vi "Scripting_FollowWireUpStream.vi"(0 "Scripting in":refnum<class "Scripting.lvclass">, 1 "StartTerminalRef":refnum<vi>, 5 "error in (no error)":errorcluster) -> (15 "FoundItems":T1[](array[typedef]), 19 "error out":errorcluster)   [LabVIEW 2016, in "Scripting.lvclass"]
uses:
  <resource>/Framework/Providers/Open_GDS/ClassProviders/Common/ScriptingFunctions/Scripting.lvclass
  <resource>/Framework/Providers/Open_GDS/ClassProviders/Common/ScriptingFunctions/Scripting_PastThroughObjectType.ctl
  <resource>/Framework/Providers/Open_GDS/ClassProviders/Common/ScriptingFunctions/Scripting_ObjectType.ctl
  <resource>/Framework/Providers/Open_GDS/ClassProviders/Common/ScriptingFunctions/Scripting.lvclass/Scripting.ctl
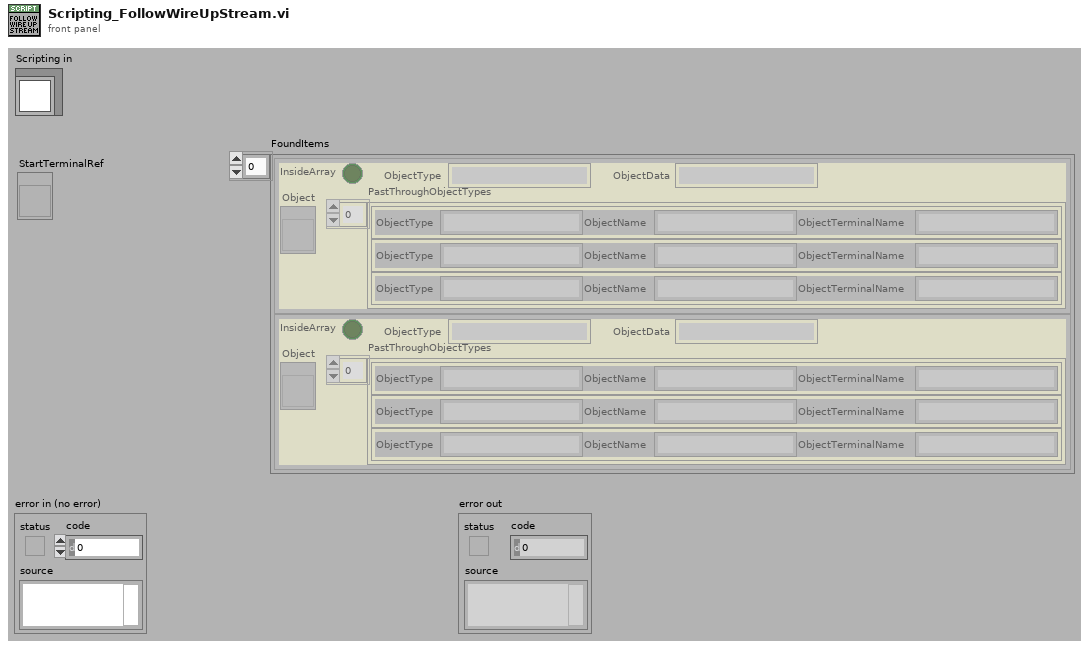
[diagram p1: front panel]
types:
  T1 = typedef "Scripting.lvclass/Scripting_PastThroughObjectType.ctl" = cluster{"Object":refnum<vi>, "InsideArray":bool, "PastThroughObjectTypes":T2[], "ObjectType":string, "ObjectData":string}
  T2 = typedef "Scripting_ObjectType.ctl" = cluster{"ObjectType":string, "ObjectName":string, "ObjectTerminalName":string}
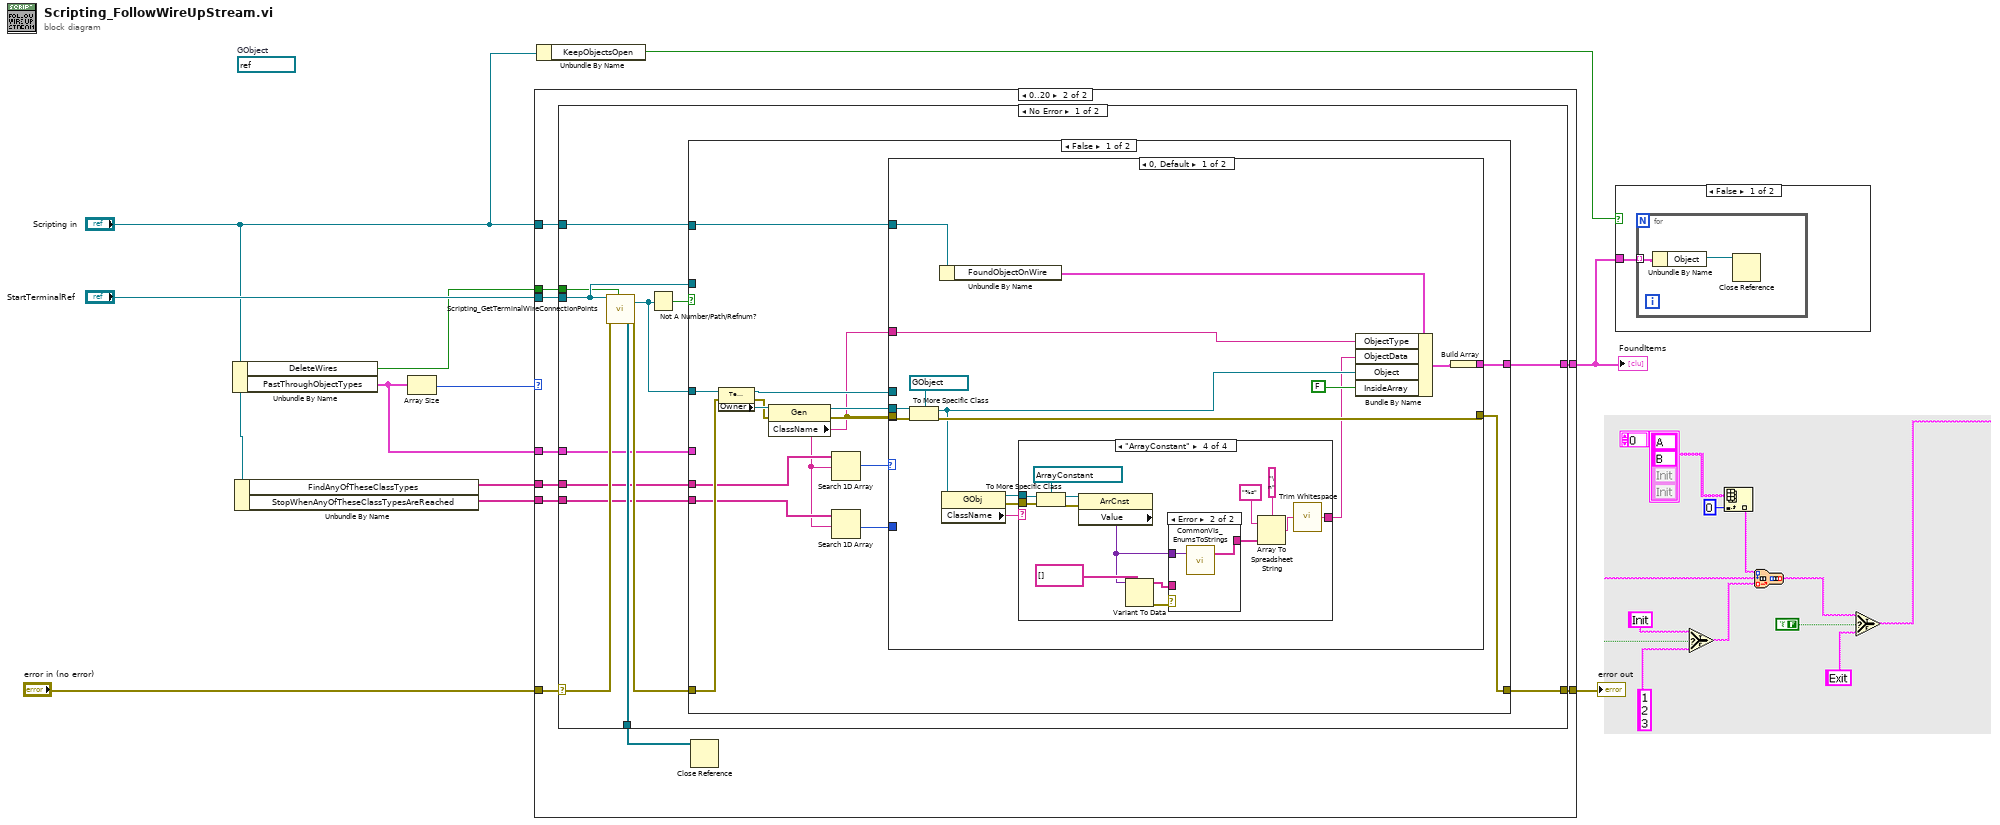
[diagram p0: block diagram]
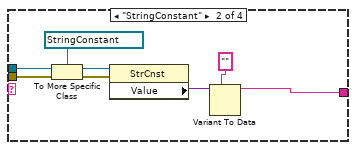
[diagram p5: hidden frame]
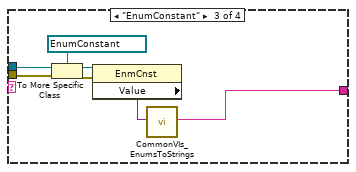
[diagram p6: hidden frame]
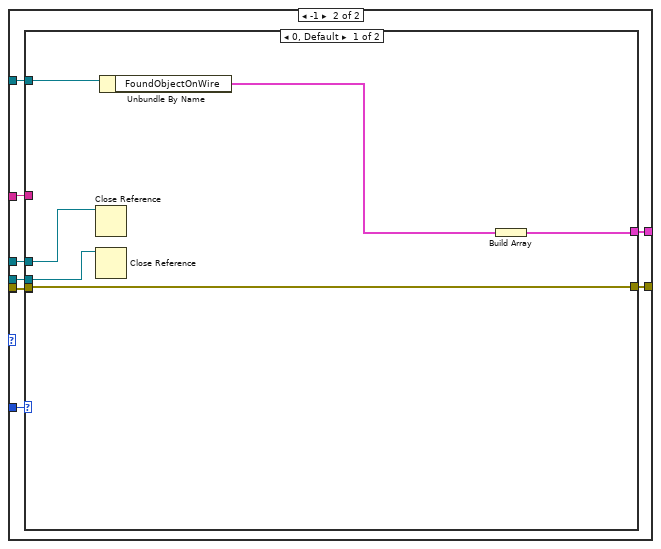
[diagram p8: hidden frame]
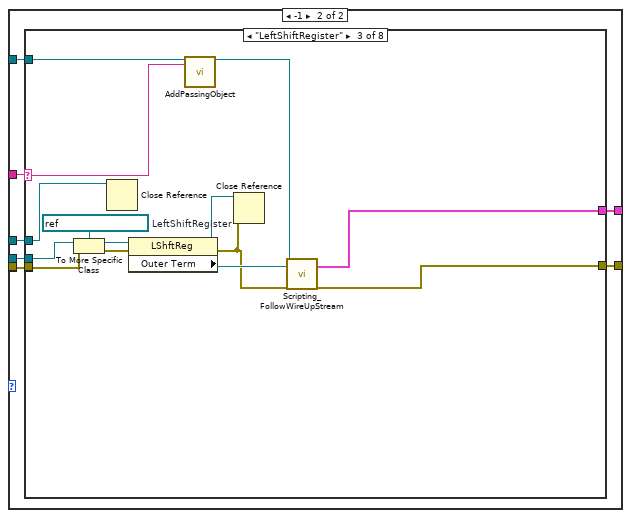
[diagram p9: hidden frame]
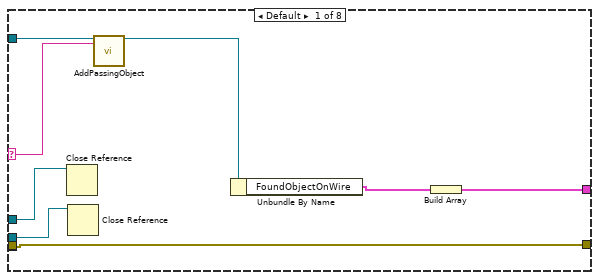
[diagram p10: hidden frame]
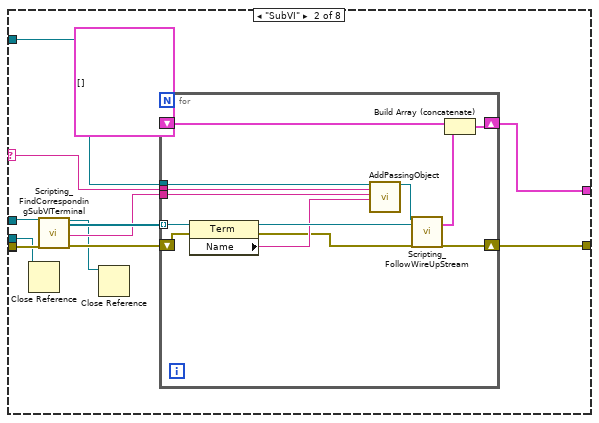
[diagram p11: hidden frame]
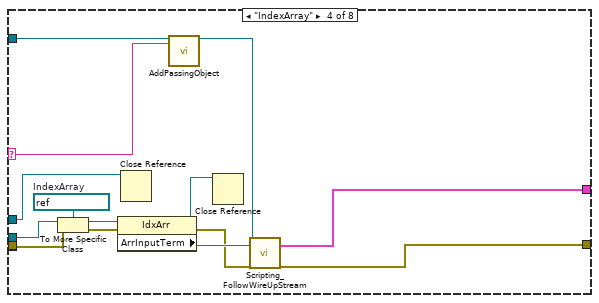
[diagram p12: hidden frame]
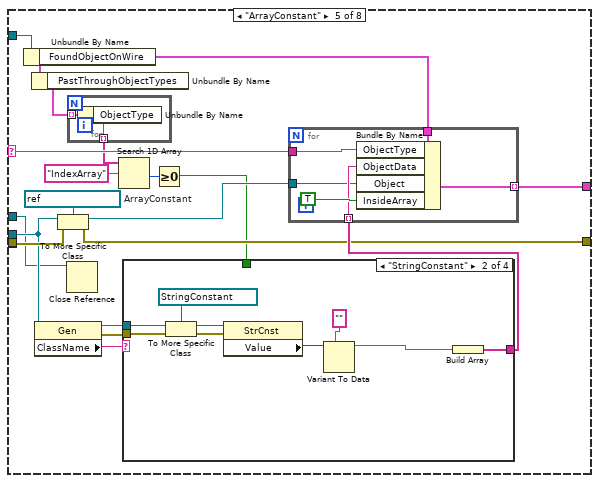
[diagram p13: hidden frame]
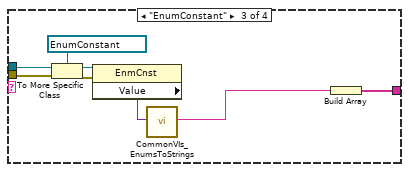
[diagram p15: hidden frame]
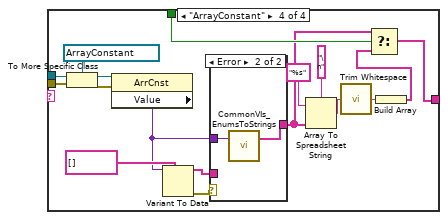
[diagram p16: hidden frame]
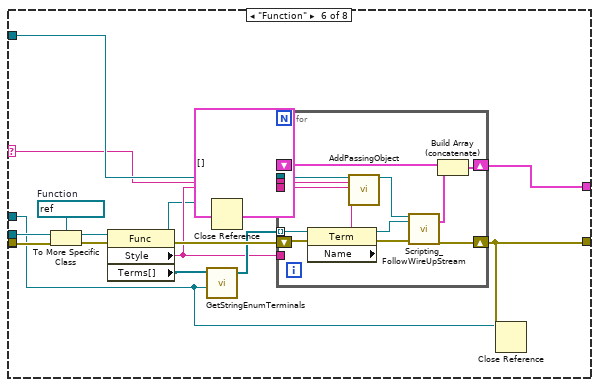
[diagram p18: hidden frame]
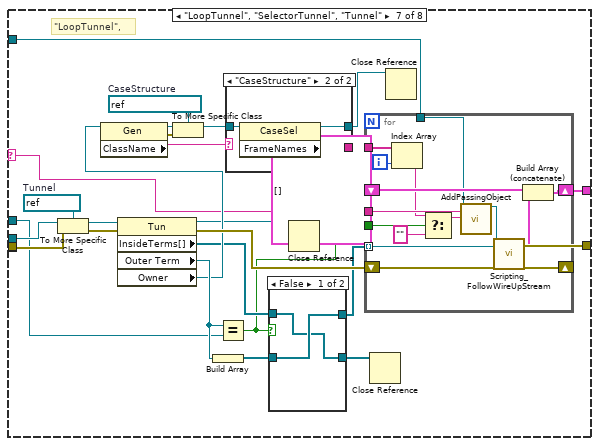
[diagram p19: hidden frame]
diagram:
  (unwired) refnum<vi> refnum  # GObject
  n1 = Unbundle By Name("Scripting in") -> ("DeleteWires"=w1:bool, "PastThroughObjectTypes"=w5:T2[])
  n2 = Unbundle By Name("Scripting in") -> ("FindAnyOfTheseClassTypes"=w8:string[], "StopWhenAnyOfTheseClassTypesAreReached"=w7:string[])
  n3 = Array Size(array=w5) -> (size(s)=w6:i32)
  n4 = case shown="0..20" w6 {
    tunnel: [w12 w22] -> w11
    tunnel: "error in (no error)" -> [w12 w21]
    tunnel: "StartTerminalRef" -> [_ w20]
    tunnel: w8 -> [_ w18]
    tunnel: w7 -> [_ w17]
    tunnel: [_ w16] -> w4
    tunnel: "Scripting in" -> [_ w15]
    tunnel: w5 -> [_ w14]
    tunnel: w1 -> [_ w13]
    frame Default {
    }
    frame 0..20 {
      n5 = case shown="No Error" w21 {
        selector: w21 -> [w31 w369]
        tunnel: [w33 w369] -> w22
        tunnel: w15 -> [w29 _]
        tunnel: w20 -> [w25 _]
        tunnel: [w35 _] -> w19
        tunnel: w18 -> [w28 _]
        tunnel: w17 -> [w27 _]
        tunnel: [w26 _] -> w16
        tunnel: w14 -> [w24 _]
        tunnel: w13 -> [w23 _]
        frame No Error {
          n6 = call <resource>:"Scripting_GetTerminalWireConnectionPoints.vi"("Term Refnum In"=w25, "error in"=w31, "RemoveWire(False)"=w23) -> ("AllWireTerminals"=w35:refnum<vi>[], "WireTermSource"=w32:refnum<vi>, "error out"=w30:errorcluster)  [unwired: 8 in, 6 out]
          n7 = Not A Number/Path/Refnum?(number/path/refnum=w32) -> (NaN/Path/Refnum?=w34:bool)
          n8 = case shown="False" w34 {
            tunnel: w30 -> [w49 w360]
            tunnel: [w47 w360] -> w33
            tunnel: w32 -> [w50 _]
            tunnel: w29 -> [w48 w355]
            tunnel: w28 -> [w46 _]
            tunnel: w27 -> [w45 _]
            tunnel: [w37 w352] -> w26
            tunnel: w25 -> [_ w354]
            tunnel: w24 -> [_ w359]
            frame False {
              n9 = property class="Term"(reference=w50, error in=w49) -> (reference out=w38:refnum<vi>, error out=w41:errorcluster, "Owner"=w42:refnum<vi>)
              n10 = property class="Gen"(reference=w42, error in=w41) -> (reference out=w39:refnum<vi>, error out=w40:errorcluster, "ClassName"=w36:string)
              n11 = Search 1D Array(1D array=w46, element=w36) -> (index of element=w44:i32)  [unwired: 1 in]
              n12 = Search 1D Array(1D array=w45, element=w36) -> (index of element=w43:i32)  [unwired: 1 in]
              n13 = case shown="0, Default" w44 {
                tunnel: w48 -> [w61 w106]
                tunnel: [w62 w105] -> w47
                tunnel: w36 -> [w56 w104]
                tunnel: w43 -> [_ w103]
                tunnel: w40 -> [w65 w102]
                tunnel: w40 -> [_ w101]
                tunnel: w39 -> [w64 w99]
                tunnel: w38 -> [_ w100]
                tunnel: [w57 w98] -> w37
                frame 0, Default {
                  n14 = To More Specific Class(target class=refnum<vi> refnum ("Object"), reference=w64, error in=w65) -> (specific class reference=w55:refnum<vi>, error out=w62:errorcluster)
                  n15 = Unbundle By Name(w61) -> ("FoundObjectOnWire"=w60:T1)
                  n16 = property class="GObj"(reference=w55) -> (reference out=w53:refnum<vi>, error out=w52:errorcluster, "ClassName"=w54:string)  [unwired: 1 in]
                  n17 = case shown="\"ArrayConstant\"" w54 {
                    tunnel: w53 -> [_ w72 w76 w87]
                    tunnel: w52 -> [_ w71 w75 w86]
                    tunnel: [_ w66 w74 w81] -> w51
                    frame Default {
                    }
                    frame "StringConstant" {
                      n18 = To More Specific Class(target class=refnum<vi> refnum ("Object"), reference=w72, error in=w71) -> (specific class reference=w70:refnum<vi>, error out=w69:errorcluster)
                      n19 = property class="StrCnst"(reference=w70, error in=w69) -> ("Value"=w68:variant)  [unwired: 2 out]
                      n20 = Variant To Data(type="" ("Class Name"), Variant=w68) -> (data=w66:string)  [unwired: 1 in, 1 out]
                    }
                    frame "EnumConstant" {
                      n21 = To More Specific Class(target class=refnum<vi> refnum ("WhileLoop"), reference=w76, error in=w75) -> (specific class reference=w79:refnum<vi>, error out=w78:errorcluster)
                      n22 = property class="EnmCnst"(reference=w79, error in=w78) -> ("Value"=w77:variant)  [unwired: 2 out]
                      n23 = call <resource>:"CommonVIs_EnumsToStrings.vi"("SingleEnumVariantIn"=w77) -> ("EnumItem"=w74:string)  [unwired: 2 in, 16 out]
                    }
                    frame "ArrayConstant" {
                      n24 = To More Specific Class(target class=refnum<vi> refnum ("WhileLoop"), reference=w87, error in=w86) -> (specific class reference=w93:refnum<vi>, error out=w92:errorcluster)
                      n25 = property class="ArrCnst"(reference=w93, error in=w92) -> ("Value"=w89:variant)  [unwired: 2 out]
                      n26 = Variant To Data(type=string[] [], Variant=w89) -> (data=w88:string[], error out=w90:errorcluster)  [unwired: 1 in]
                      n27 = case shown="Error" w90 {
                        tunnel: w89 -> [_ w97]
                        tunnel: w88 -> [w95 _]
                        tunnel: [w95 w96] -> w85
                        frame No Error {
                        }
                        frame Error {
                          n28 = call <resource>:"CommonVIs_EnumsToStrings.vi"("ArrayEnumVariantIn"=w97) -> ("EnumItems(string)"=w96:string[])  [unwired: 2 in, 16 out]
                        }
                      }
                      n29 = Array To Spreadsheet String(delimiter (Tab)="\n", array=w85, 3:"%s" ("format string")) -> (spreadsheet string=w82:string)
                      n30 = call <vilib>:"Trim Whitespace.vi"("string"=w82) -> ("trimmed string"=w81:string)  [unwired: 1 in]
                    }
                  }
                  n31 = Bundle By Name(cluster=w60, "ObjectType"=w56, "ObjectData"=w51, "Object"=w55, "InsideArray"=FALSE) -> (w58:T1)
                  n32 = Build Array(w58) -> (w57:T1[])
                }
                frame -1 {
                  n33 = case shown="0, Default" w103 {
                    tunnel: w106 -> [w109 w120]
                    tunnel: [w112 w119] -> w105
                    tunnel: w104 -> [_ w118]
                    tunnel: w102 -> [w112 w117]
                    tunnel: w101 -> [_ w116]
                    tunnel: w100 -> [w111 w115]
                    tunnel: w99 -> [w110 w114]
                    tunnel: [w107 w113] -> w98
                    frame 0, Default {
                      n34 = Close Reference(reference=w111) -> ()  [unwired: 1 in, 1 out]
                      n35 = Close Reference(reference=w110) -> ()  [unwired: 1 in, 1 out]
                      n36 = Unbundle By Name(w109) -> ("FoundObjectOnWire"=w108:T1)
                      n37 = Build Array(w108) -> (w107:T1[])
                    }
                    frame -1 {
                      n38 = case shown="\"LeftShiftRegister\"" w118 {
                        selector: w118 -> [w126 w132 w157 w169 w190 w249 w281 w332]
                        tunnel: w120 -> [w127 w133 w159 w171 w192 w250 w282 w333]
                        tunnel: [w128 w140 w162 w174 w188 w246 w296 w338] -> w119
                        tunnel: w117 -> [w128 _ w166 w180 w199 w260 w300 w341]
                        tunnel: w116 -> [_ w137 _ _ _ _ _ _]
                        tunnel: w115 -> [w125 w136 w153 w167 w181 w245 w290 w331]
                        tunnel: w114 -> [w124 w129 w161 w173 w193 w256 w295 w337]
                        tunnel: [w121 w134 w160 w172 w197 w254 w293 w335] -> w113
                        frame Default {
                          n39 = Close Reference(reference=w125) -> ()  [unwired: 1 in, 1 out]
                          n40 = Close Reference(reference=w124) -> ()  [unwired: 1 in, 1 out]
                          n41 = call <resource>:"AddPassingObject.vi"("object in"=w127, "PassingThroughObject"=w126) -> ("object out"=w123:refnum<class "Scripting.lvclass">)  [unwired: 16 in, 1 out]
                          n42 = Unbundle By Name(w123) -> ("FoundObjectOnWire"=w122:T1)
                          n43 = Build Array(w122) -> (w121:T1[])
                        }
                        frame "SubVI" {
                          n44 = Close Reference(reference=w129) -> ()  [unwired: 1 in, 1 out]
                          n45 = call <resource>:"Scripting_FindCorrespondingSubVITerminal.vi"("SubVITerminalIn"=w136, "error in"=w137) -> ("SubVITerminalIn Dub"=w130:refnum<vi>, "SubVITerminalOut"=w138:refnum<vi>[], "VI Name"=w131:string, "error out"=w139:errorcluster)  [unwired: 11 in, 3 out]
                          n46 = Close Reference(reference=w130) -> ()  [unwired: 1 in, 1 out]
                          n47 = for {
                            tunnel: w138 -> [w143] mode=indexing
                            shift-right: [w152] -> w140
                            shift-left: w139 -> [w144]
                            shift-right: [w150] -> w134
                            shift-left: T1[] [] ("FoundItems") -> [w151]
                            tunnel: w133 -> [w148]
                            tunnel: w132 -> [w146]
                            tunnel: w131 -> [w145]
                            n48 = property class="Term"(reference=w143, error in=w144) -> (error out=w141:errorcluster, "Name"=w142:string)  [unwired: 1 out]
                            n49 = call <resource>:"AddPassingObject.vi"("object in"=w148, "PassingThroughObject"=w146, "PassingThroughObjectName"=w145, "TerminalName"=w142) -> ("object out"=w147:refnum<class "Scripting.lvclass">)  [unwired: 14 in, 1 out]
                            n50 = call-dynamic "Scripting_FollowWireUpStream.vi"("Scripting in"=w147, "StartTerminalRef"=w143, "error in (no error)"=w141) -> ("FoundItems"=w149:T1[], "error out"=w152:errorcluster)  [unwired: 15 in]
                            n51 = Build Array (concatenate)(w151, w149) -> (w150:T1[])
                          }
                        }
                        frame "LeftShiftRegister" {
                          w165 = refnum<vi> refnum  # LeftShiftRegister
                          n52 = To More Specific Class(target class=w165, reference=w161, error in=w166) -> (specific class reference=w154:refnum<vi>, error out=w163:errorcluster)
                          n53 = Close Reference(reference=w153) -> ()  [unwired: 1 in, 1 out]
                          n54 = property class="LShftReg"(reference=w154, error in=w163) -> (reference out=w156:refnum<vi>, error out=w155:errorcluster, "Outer Term"=w164:refnum<vi>)
                          n55 = call <resource>:"AddPassingObject.vi"("object in"=w159, "PassingThroughObject"=w157) -> ("object out"=w158:refnum<class "Scripting.lvclass">)  [unwired: 16 in, 1 out]
                          n56 = Close Reference(reference=w156, error in (no error)=w155) -> ()  [unwired: 1 out]
                          n57 = call-dynamic "Scripting_FollowWireUpStream.vi"("Scripting in"=w158, "StartTerminalRef"=w164, "error in (no error)"=w155) -> ("FoundItems"=w160:T1[], "error out"=w162:errorcluster)  [unwired: 15 in]
                        }
                        frame "IndexArray" {
                          w179 = refnum<vi> refnum  # IndexArray
                          n58 = To More Specific Class(target class=w179, reference=w173, error in=w180) -> (specific class reference=w178:refnum<vi>, error out=w176:errorcluster)
                          n59 = property class="IdxArr"(reference=w178, error in=w176) -> (reference out=w168:refnum<vi>, error out=w175:errorcluster, "ArrInputTerm"=w177:refnum<vi>)
                          n60 = Close Reference(reference=w167) -> ()  [unwired: 1 in, 1 out]
                          n61 = call <resource>:"AddPassingObject.vi"("object in"=w171, "PassingThroughObject"=w169) -> ("object out"=w170:refnum<class "Scripting.lvclass">)  [unwired: 16 in, 1 out]
                          n62 = Close Reference(reference=w168) -> ()  [unwired: 1 in, 1 out]
                          n63 = call-dynamic "Scripting_FollowWireUpStream.vi"("Scripting in"=w170, "StartTerminalRef"=w177, "error in (no error)"=w175) -> ("FoundItems"=w172:T1[], "error out"=w174:errorcluster)  [unwired: 15 in]
                        }
                        frame "ArrayConstant" {
                          w198 = refnum<vi> refnum  # ArrayConstant
                          n64 = Unbundle By Name(w192) -> ("FoundObjectOnWire"=w187:T1)
                          n65 = Unbundle By Name(w187) -> ("PastThroughObjectTypes"=w186:T2[])
                          n66 = property class="Gen"(reference=w193) -> (reference out=w195:refnum<vi>, error out=w194:errorcluster, "ClassName"=w196:string)  [unwired: 1 in]
                          n67 = To More Specific Class(target class=w198, reference=w193, error in=w199) -> (specific class reference=w189:refnum<vi>, error out=w188:errorcluster)
                          n68 = Close Reference(reference=w181) -> ()  [unwired: 1 in, 1 out]
                          n69 = for {
                            tunnel: w186 -> [w201] mode=indexing
                            tunnel: [w200] -> w185 mode=indexing
                            n70 = Unbundle By Name(w201) -> ("ObjectType"=w200:string)
                          }
                          n71 = Search 1D Array(1D array=w185, element="IndexArray") -> (index of element=w183:i32)  [unwired: 1 in]
                          n72 = Greater Or Equal To 0?(x=w183) -> (x >= 0?=w182:bool)
                          n73 = case shown="\"StringConstant\"" w196 {
                            tunnel: w195 -> [_ w215 w220 w234]
                            tunnel: w194 -> [_ w214 w219 w233]
                            tunnel: [_ w208 w217 w225] -> w191
                            tunnel: w182 -> [_ _ _ w228]
                            frame Default {
                            }
                            frame "StringConstant" {
                              n74 = To More Specific Class(target class=refnum<vi> refnum ("Object"), reference=w215, error in=w214) -> (specific class reference=w213:refnum<vi>, error out=w212:errorcluster)
                              n75 = property class="StrCnst"(reference=w213, error in=w212) -> ("Value"=w211:variant)  [unwired: 2 out]
                              n76 = Variant To Data(type="" ("Class Name"), Variant=w211) -> (data=w209:string)  [unwired: 1 in, 1 out]
                              n77 = Build Array(w209) -> (w208:string[])
                            }
                            frame "EnumConstant" {
                              n78 = To More Specific Class(target class=refnum<vi> refnum ("WhileLoop"), reference=w220, error in=w219) -> (specific class reference=w223:refnum<vi>, error out=w222:errorcluster)
                              n79 = property class="EnmCnst"(reference=w223, error in=w222) -> ("Value"=w221:variant)  [unwired: 2 out]
                              n80 = call <resource>:"CommonVIs_EnumsToStrings.vi"("SingleEnumVariantIn"=w221) -> ("EnumItem"=w218:string)  [unwired: 2 in, 16 out]
                              n81 = Build Array(w218) -> (w217:string[])
                            }
                            frame "ArrayConstant" {
                              n82 = To More Specific Class(target class=refnum<vi> refnum ("WhileLoop"), reference=w234, error in=w233) -> (specific class reference=w240:refnum<vi>, error out=w239:errorcluster)
                              n83 = property class="ArrCnst"(reference=w240, error in=w239) -> ("Value"=w236:variant)  [unwired: 2 out]
                              n84 = Variant To Data(type=string[] [], Variant=w236) -> (data=w235:string[], error out=w237:errorcluster)  [unwired: 1 in]
                              n85 = case shown="Error" w237 {
                                tunnel: w236 -> [_ w244]
                                tunnel: w235 -> [w242 _]
                                tunnel: [w242 w243] -> w227
                                frame No Error {
                                }
                                frame Error {
                                n86 = call <resource>:"CommonVIs_EnumsToStrings.vi"("ArrayEnumVariantIn"=w244) -> ("EnumItems(string)"=w243:string[])  [unwired: 2 in, 16 out]
                                }
                              }
                              n87 = Array To Spreadsheet String(delimiter (Tab)="\n", array=w227, 3:"%s" ("format string")) -> (spreadsheet string=w230:string)
                              n88 = call <vilib>:"Trim Whitespace.vi"("string"=w230) -> ("trimmed string"=w229:string)  [unwired: 1 in]
                              n89 = Build Array(w229) -> (w226:string[])
                              n90 = Select(t=w227, s=w228, f=w226) -> (s? t:f=w225:string[])
                            }
                          }
                          n91 = for {
                            tunnel: w187 -> [w207]
                            tunnel: [w202] -> w197 mode=indexing
                            tunnel: w191 -> [w205] mode=indexing
                            tunnel: w190 -> [w204]
                            tunnel: w189 -> [w203]
                            n92 = Bundle By Name(cluster=w207, "ObjectType"=w204, "ObjectData"=w205, "Object"=w203, "InsideArray"=TRUE) -> (w202:T1)
                          }
                        }
                        frame "Function" {
                          w259 = refnum<vi> refnum  # Function
                          n93 = To More Specific Class(target class=w259, reference=w256, error in=w260) -> (specific class reference=w258:refnum<vi>, error out=w257:errorcluster)
                          n94 = property class="Func"(reference=w258, error in=w257) -> (reference out=w247:refnum<vi>, error out=w253:errorcluster, "Style"=w248:string, "Terms[]"=w251:refnum<vi>[])
                          n95 = call <resource>:"GetStringEnumTerminals.vi"("WireTerminal"=w245, "Terms[]"=w251) -> ("Array"=w252:refnum<vi>[])  [unwired: 8 in, 1 out]
                          n96 = Close Reference(reference=w247) -> ()  [unwired: 1 in, 1 out]
                          n97 = for {
                            tunnel: w252 -> [w262] mode=indexing
                            shift-right: [w273] -> w246
                            shift-left: w253 -> [w265]
                            shift-right: [w270] -> w254
                            shift-left: T1[] [] ("FoundItems") -> [w272]
                            tunnel: w248 -> [_]
                            tunnel: w250 -> [w269]
                            tunnel: w249 -> [w267]
                            tunnel: w248 -> [w266]
                            n98 = property class="Term"(reference=w262, error in=w265) -> (reference out=w261:refnum<vi>, error out=w263:errorcluster, "Name"=w264:string)
                            n99 = call <resource>:"AddPassingObject.vi"("object in"=w269, "PassingThroughObject"=w267, "PassingThroughObjectName"=w266, "TerminalName"=w264) -> ("object out"=w268:refnum<class "Scripting.lvclass">)  [unwired: 14 in, 1 out]
                            n100 = call-dynamic "Scripting_FollowWireUpStream.vi"("Scripting in"=w268, "StartTerminalRef"=w261, "error in (no error)"=w263) -> ("FoundItems"=w271:T1[], "error out"=w273:errorcluster)  [unwired: 15 in]
                            n101 = Build Array (concatenate)(w272, w271) -> (w270:T1[])
                          }
                          n102 = Close Reference(reference=w245, error in (no error)=w246) -> ()  [unwired: 1 out]
                        }
                        frame "LoopTunnel", "SelectorTunnel", "Tunnel" {
                          w285 = refnum<vi> refnum  # CaseStructure
                          w299 = refnum<vi> refnum  # Tunnel
                          # "\"LoopTunnel\","
                          n103 = To More Specific Class(target class=w299, reference=w295, error in=w300) -> (specific class reference=w291:refnum<vi>, error out=w298:errorcluster)
                          n104 = property class="Tun"(reference=w291, error in=w298) -> (reference out=w275:refnum<vi>, error out=w297:errorcluster, "InsideTerms[]"=w278:refnum<vi>[], "Outer Term"=w292:refnum<vi>, "Owner"=w288:refnum<vi>)
                          n105 = property class="Gen"(reference=w288) -> (reference out=w287:refnum<vi>, error out=w286:errorcluster, "ClassName"=w284:string)  [unwired: 1 in]
                          n106 = To More Specific Class(target class=w285, reference=w287, error in=w286) -> (specific class reference=w283:refnum<vi>)  [unwired: 1 out]
                          n107 = Build Array(w292) -> (w279:refnum<vi>[])
                          n108 = Equal?(x=w292, y=w290) -> (x = y?=w274:bool)
                          n109 = case shown="\"CaseStructure\"" w284 {
                            tunnel: w283 -> [w305 w308]
                            tunnel: [_ w307] -> w280
                            tunnel: [w305 w306] -> w276
                            frame Default {
                            }
                            frame "CaseStructure" {
                              n110 = property class="CaseSel"(reference=w308) -> (reference out=w306:refnum<vi>, "FrameNames"=w307:string[])  [unwired: 1 in, 1 out]
                            }
                          }
                          n111 = case shown="False" w274 {
                            tunnel: [w302 w304] -> w289
                            tunnel: w279 -> [w302 w303]
                            tunnel: w278 -> [w301 w304]
                            tunnel: [w301 w303] -> w277
                            frame False {
                            }
                            frame True {
                            }
                          }
                          n112 = Close Reference(reference=w275) -> ()  [unwired: 1 in, 1 out]
                          n113 = for {
                            tunnel: w289 -> [w323] mode=indexing
                            shift-right: [w321] -> w296
                            shift-left: w297 -> [w322]
                            shift-right: [w318] -> w293
                            shift-left: T1[] [] ("FoundItems") -> [w320]
                            tunnel: w282 -> [w317]
                            tunnel: w281 -> [w315]
                            tunnel: w280 -> [w314]
                            tunnel: w274 -> [w310]
                            i -> [w313]
                            n114 = Index Array(array=w314, index=w313) -> (element=w311:string)
                            n115 = Select(t=w311, s=w310, f="") -> (s? t:f=w312:string)
                            n116 = call <resource>:"AddPassingObject.vi"("object in"=w317, "PassingThroughObject"=w315, "PassingThroughObjectName"=w312) -> ("object out"=w316:refnum<class "Scripting.lvclass">)  [unwired: 15 in, 1 out]
                            n117 = call-dynamic "Scripting_FollowWireUpStream.vi"("Scripting in"=w316, "StartTerminalRef"=w323, "error in (no error)"=w322) -> ("FoundItems"=w319:T1[], "error out"=w321:errorcluster)  [unwired: 15 in]
                            n118 = Build Array (concatenate)(w320, w319) -> (w318:T1[])
                          }
                          n119 = Close Reference(reference=w277) -> ()  [unwired: 1 in, 1 out]
                          n120 = Close Reference(reference=w276) -> ()  [unwired: 1 in, 1 out]
                        }
                        frame "Comparison" {
                          w340 = refnum<vi> refnum  # Comparison
                          n121 = To More Specific Class(target class=w340, reference=w337, error in=w341) -> (specific class reference=w334:refnum<vi>, error out=w339:errorcluster)
                          n122 = property class="Comp"(reference=w334, error in=w339) -> (reference out=w326:refnum<vi>, error out=w325:errorcluster, "Terms[]"=w330:refnum<vi>[])
                          n123 = Search 1D Array(1D array=w330, element=w331) -> (index of element=w329:i32)  [unwired: 1 in]
                          n124 = Delete From Array(array=w330, index=w329) -> (deleted portion=w328:refnum<vi>, array with subset deleted=w327:refnum<vi>[])  [unwired: 1 in]
                          n125 = Close Reference(reference=w326, error in (no error)=w325) -> (error out=w324:errorcluster)
                          n126 = Close Reference(reference=w328) -> ()  [unwired: 1 in, 1 out]
                          n127 = for {
                            tunnel: w327 -> [w350] mode=indexing
                            shift-right: [w348] -> w338
                            shift-left: w324 -> [w349]
                            shift-right: [w345] -> w335
                            shift-left: T1[] [] ("FoundItems") -> [w347]
                            tunnel: w333 -> [w344]
                            tunnel: w332 -> [w342]
                            n128 = call <resource>:"AddPassingObject.vi"("object in"=w344, "PassingThroughObject"=w342) -> ("object out"=w343:refnum<class "Scripting.lvclass">)  [unwired: 16 in, 1 out]
                            n129 = call-dynamic "Scripting_FollowWireUpStream.vi"("Scripting in"=w343, "StartTerminalRef"=w350, "error in (no error)"=w349) -> ("FoundItems"=w346:T1[], "error out"=w348:errorcluster)  [unwired: 15 in]
                            n130 = Build Array (concatenate)(w347, w346) -> (w345:T1[])
                          }
                        }
                      }
                    }
                  }
                }
              }
            }
            frame True {
              n131 = Delete From Array(array=w359) -> (deleted portion=w358:T2)  [unwired: 2 in, 1 out]
              n132 = Unbundle By Name(w358) -> ("ObjectType"=w357:string)
              n133 = Equal?(x="SelectorTunnel", y=w357) -> (x = y?=w351:bool)
              n134 = case shown="False" w351 {
                tunnel: w355 -> [_ w365]
                tunnel: w354 -> [w361 w364]
                tunnel: [_ w363] -> w353
                frame False {
                  n135 = Close Reference(reference=w361) -> ()  [unwired: 1 in, 1 out]
                }
                frame True {
                  n136 = Unbundle By Name(w365) -> ("FoundObjectOnWire"=w368:T1)
                  n137 = Bundle By Name(cluster=w368, "ObjectType"="UseDefault", "ObjectData"="\"\"", "Object"=w364, "InsideArray"=FALSE) -> (w363:T1)
                }
              }
              n138 = Build Array(w353) -> (w352:T1[])
            }
          }
        }
        frame Error {
        }
      }
      n139 = Close Reference(reference=w19) -> ()  [unwired: 1 in, 1 out]
    }
  }
  "error out" <- w11
  "FoundItems" <- w4
  n140 = Unbundle By Name("Scripting in") -> ("KeepObjectsOpen"=w2:bool)
  n141 = case shown="False" w2 {
    tunnel: w4 -> [w370 _]
    frame False {
      n142 = for {
        tunnel: w370 -> [w372] mode=indexing
        n143 = Unbundle By Name(w372) -> ("Object"=w371:refnum<vi>)
        n144 = Close Reference(reference=w371) -> ()  [unwired: 1 in, 1 out]
      }
    }
    frame True {
    }
  }
